vi "test_harness_HM_times_x_preload.vi"() -> ()   [LabVIEW 2017]
uses:
  fgm_pipiline_mine/x_vec_type.ctl
  quadProgControls/x_qp_scalar.ctl
  <vilib>/rvi/Memory/Memory_Emulation/nirvimemoryFastEmulation.vi
  <vilib>/rvi/Memory/Memory_Emulation/nirvimemoryEmulation.vi
  <vilib>/rvi/Emulation/niFpgaEmulationIsFPGAContextNoSignature.vi
  <vilib>/rvi/DataTransferAndStorage/Container/Common/niFpgaContainerGetUniqueNameForEmu.vi
  <vilib>/rvi/Emulation/niFpgaProcessEmulError.vi
  <vilib>/rvi/Emulation/niFpgaSctlEmulationGetInTimedLoop.vi
  <vilib>/rvi/errors/nirviReportUnexpectedCaseInternalError (U32).vi
  <vilib>/rvi/DataTransferAndStorage/Container/XNode/niFpgaContainer.xnode
panel:
  in  "x_vec":T1=[0.6000000238418579, 0.6000000238418579, -0.5999999940395355, -0.5999999940395355, 0.6000000238418579, 0.6000000238418579, 0.6000000238418579, 0.6000000238418579, -0.5999999940395355, 0.6000000238418579, -0.5999999940395355, -4.0, 0.0, 0.0, 0.0, 0.0, 0.0, 0.0, 0.0, 0.0, 0.0, 0.0, 0.0, 0.0, 0.0]
  in  "Ncol":u16
  in  "Ns":u16
  in  "nuN_mpc":u16
  in  "big_mat_data":fxp<+/-,32,3>[](array[numeric])=[0.0, 0.0, 0.0, 0.0, 0.0, 0.0, 0.0, 0.0, 0.0, 0.0, 0.0, 0.0]
  out "preload result":fxp<+/-,32,2>[](array[numeric]) format="%.31g"
  out "primary result":fxp<+/-,32,2>[](array[numeric]) format="%.31g"
  in  "primary_write_addr":u16
  in  "preload_vec":fxp<+/-,32,3>[](array[numeric])=[0.0, 0.0, 0.0, 0.0, 0.0, 0.0, 0.0, 0.0, 0.0, 0.0, 0.0, 0.0]
  in  "preload_addr":u16
  in  "StartIndex":u16
  out "A*x":fxp<+/-,32,3>[](array[numeric])
  in  "SLMAX":fxp<+/-,18,5>
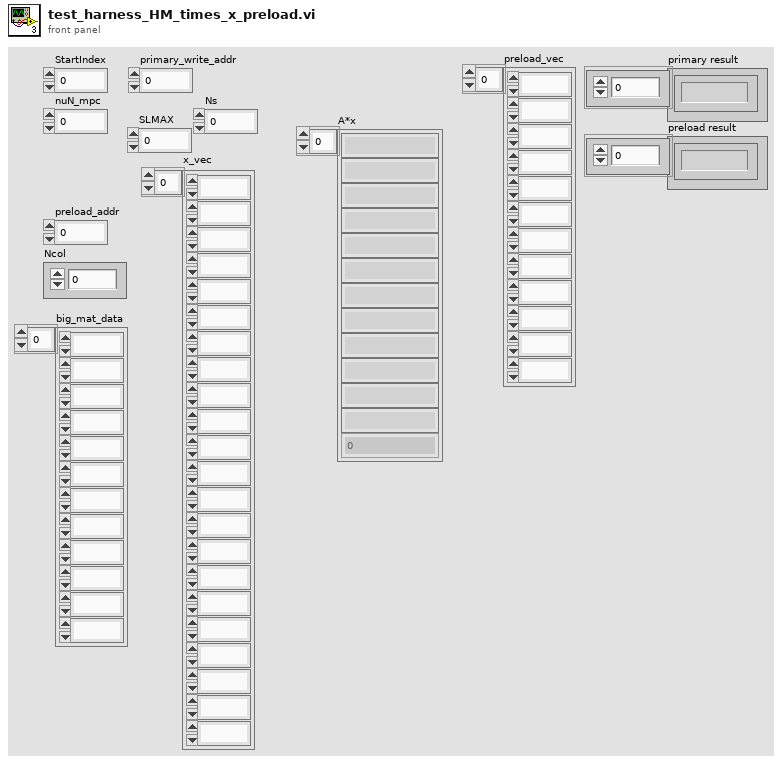
[diagram p1: front panel]
types:
  T1 = typedef "x_vec_type.ctl" = T2[]
  T2 = typedef "x_qp_scalar.ctl" = fxp<+/-,32,6>
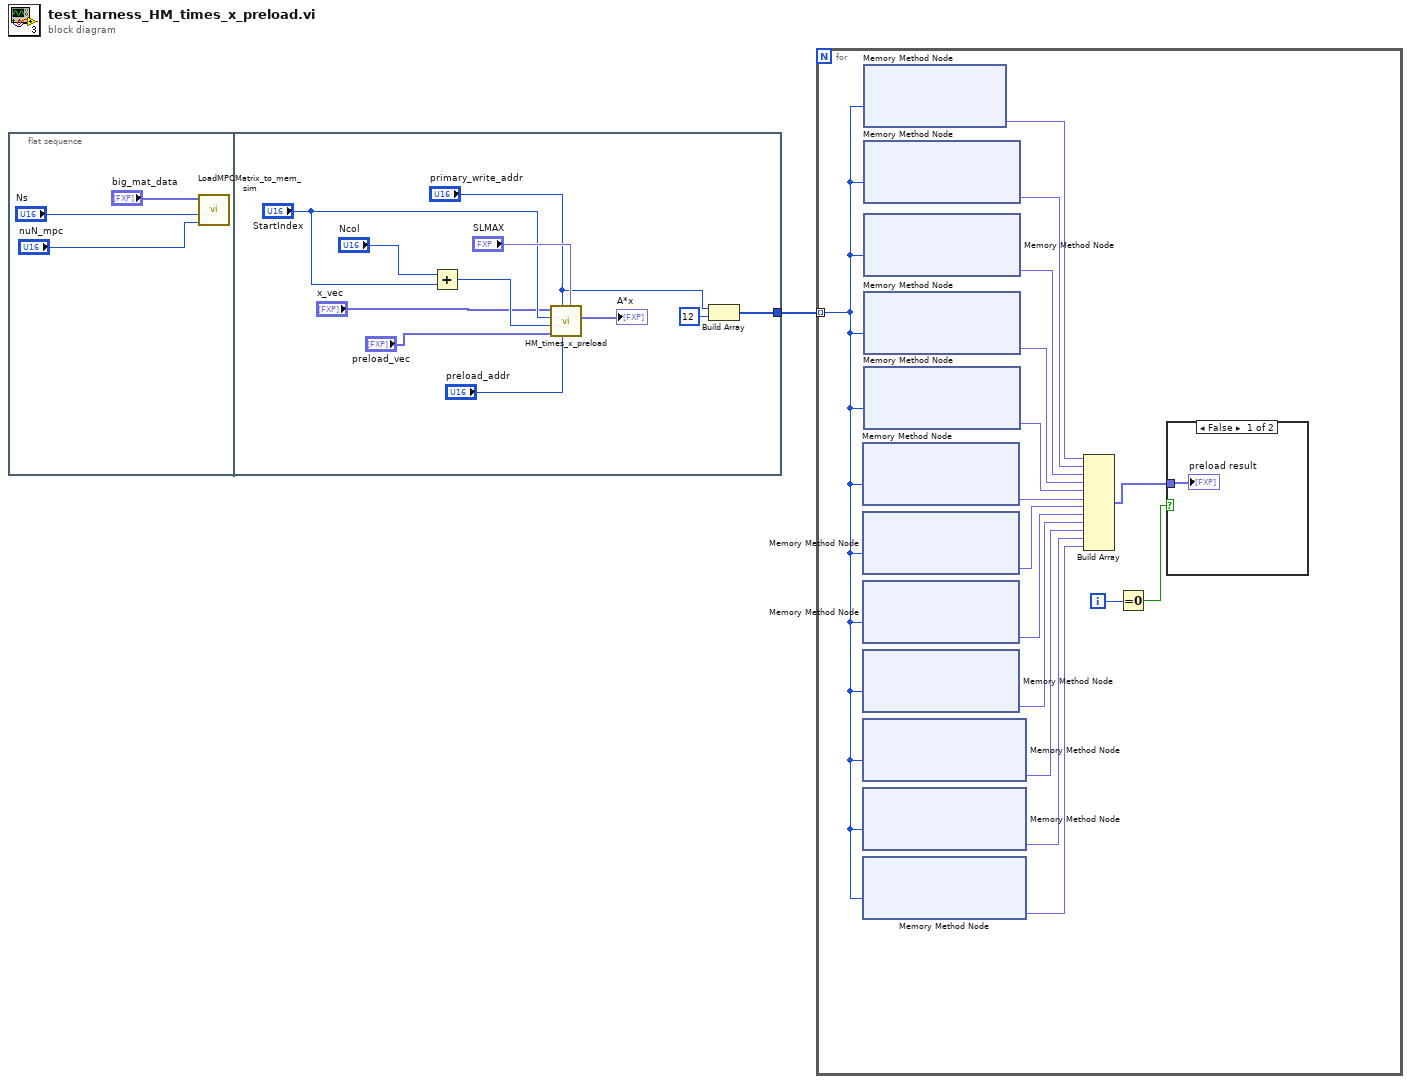
[diagram p0: block diagram]
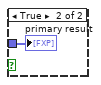
[diagram p2: hidden frame]
diagram:
  n1 = flat-sequence {
    tunnel: [w10] -> w1
    frame #0 {
      n2 = call "LoadMPCMatrix_to_mem_sim.vi"("nuN_mpc"="nuN_mpc", "Ns"="Ns", "big_mat_data"="big_mat_data") -> ()  [unwired: 9 in]
    }
    frame #1 {
      n3 = Add(x="Ncol", y="StartIndex") -> (x+y=w7:u16)
      n4 = call "HM_times_x_preload.vi"("SLMAX"="SLMAX", "preload_addr"="preload_addr", "primary_write_addr"="primary_write_addr", "preload_vec"="preload_vec", "Ns+StartIndex"=w7, "StartIndex"="StartIndex", "x_vec"="x_vec") -> ("A*x"=→"A*x":fxp<+/-,32,3>[])  [unwired: 2 in, 2 out]
      n5 = Build Array("primary_write_addr", u16 12 ("element")) -> (w10:u16[])
    }
  }
  n6 = for {
    tunnel: w1 -> [w31] mode=indexing
    i -> [w16]
    n7 = xnode ("Memory Method Node")("Address"=w31) -> ("Data"=w25:fxp<+/-,32,2>)  [unwired: 1 in, 1 out]
    n8 = xnode ("Memory Method Node")("Address"=w31) -> ("Data"=w24:fxp<+/-,32,2>)  [unwired: 1 in, 1 out]
    n9 = xnode ("Memory Method Node")("Address"=w31) -> ("Data"=w23:fxp<+/-,32,2>)  [unwired: 1 in, 1 out]
    n10 = xnode ("Memory Method Node")("Address"=w31) -> ("Data"=w22:fxp<+/-,32,2>)  [unwired: 1 in, 1 out]
    n11 = xnode ("Memory Method Node")("Address"=w31) -> ("Data"=w21:fxp<+/-,32,2>)  [unwired: 1 in, 1 out]
    n12 = xnode ("Memory Method Node")("Address"=w31) -> ("Data"=w20:fxp<+/-,32,2>)  [unwired: 1 in, 1 out]
    n13 = xnode ("Memory Method Node")("Address"=w31) -> ("Data"=w19:fxp<+/-,32,2>)  [unwired: 1 in, 1 out]
    n14 = xnode ("Memory Method Node")("Address"=w31) -> ("Data"=w30:fxp<+/-,32,2>)  [unwired: 1 in, 1 out]
    n15 = xnode ("Memory Method Node")("Address"=w31) -> ("Data"=w29:fxp<+/-,32,2>)  [unwired: 1 in, 1 out]
    n16 = xnode ("Memory Method Node")("Address"=w31) -> ("Data"=w28:fxp<+/-,32,2>)  [unwired: 1 in, 1 out]
    n17 = xnode ("Memory Method Node")("Address"=w31) -> ("Data"=w27:fxp<+/-,32,2>)  [unwired: 1 in, 1 out]
    n18 = xnode ("Memory Method Node")("Address"=w31) -> ("Data"=w26:fxp<+/-,32,2>)  [unwired: 1 in, 1 out]
    n19 = Build Array(w30, w29, w28, w27, w26, w25, w24, w23, w22, w21, w20, w19) -> (w17:fxp<+/-,32,2>[])
    n20 = Equal To 0?(x=w16) -> (x = 0?=w18:bool)
    n21 = case shown="False" w18 {
      tunnel: w17 -> [w32 w33]
      frame False {
        "preload result" <- w32
      }
      frame True {
        "primary result" <- w33
      }
    }
  }
